vi "exp3p2.vi"() -> ()   [LabVIEW 2019]
uses:
  <vilib>/sound2/lvsound2.llb/Sound Data Format.ctl
  <vilib>/sound2/lvsound2.llb/Sampling Mode.ctl
  <vilib>/Analysis/2dsp.llb/Power Spectrum (DBL).vi
  <vilib>/sound2/lvsound2.llb/Sound Output Set Volume (Single).vi
  <vilib>/sound2/lvsound2.llb/Sound Output Write (DBL Single).vi
  <vilib>/Analysis/NI_AALPro.lvlib
panel:
  in  "sample mode":T1=1 items=["Finite Samples", "Continuous Samples"]
  in  "Volume":dbl(slide) scale=0.0..100.0
  in  "sound format":T2={"sample rate (S/s)"=22050.0, "number of channels"=2, "bits per sample"=16}
  in  "device ID":u32
  out "SNR (dB)":dbl
  out "Frequency Estimate (Hz)":dbl
  out "Frequency Domain Waveform":waveform(dbl)(graph)
  out "Time Domain Waveform":waveform(dbl)(graph)
  in  "Noise Std":dbl
  in  "Frequency Deviation (Hz)":dbl
  in  "stop":bool
  in  "Sampling Frequency":dbl
  in  "AWGN":bool
  in  "phase":dbl format="%0.2f"
  in  "frequency":dbl=1.0 format="%0.2f"
  in  "amplitude":dbl=1.0 format="%0.2f"
  in  "Frequency Hopping":bool
  in  "Number of Samples":i32
  in  "Square vs Sine":bool
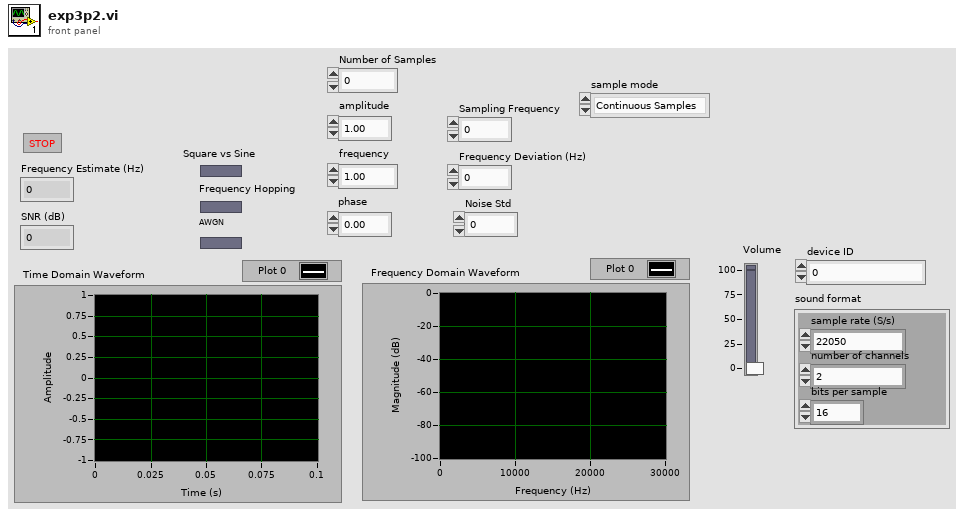
[diagram p1: front panel]
types:
  T1 = typedef "Sampling Mode.ctl" = i32
  T2 = typedef "Sound Data Format.ctl" = cluster{"sample rate (S/s)":dbl, "number of channels":i32, "bits per sample":i32}
  T3 = typedef "Sound Output Task ID.ctl" = u32
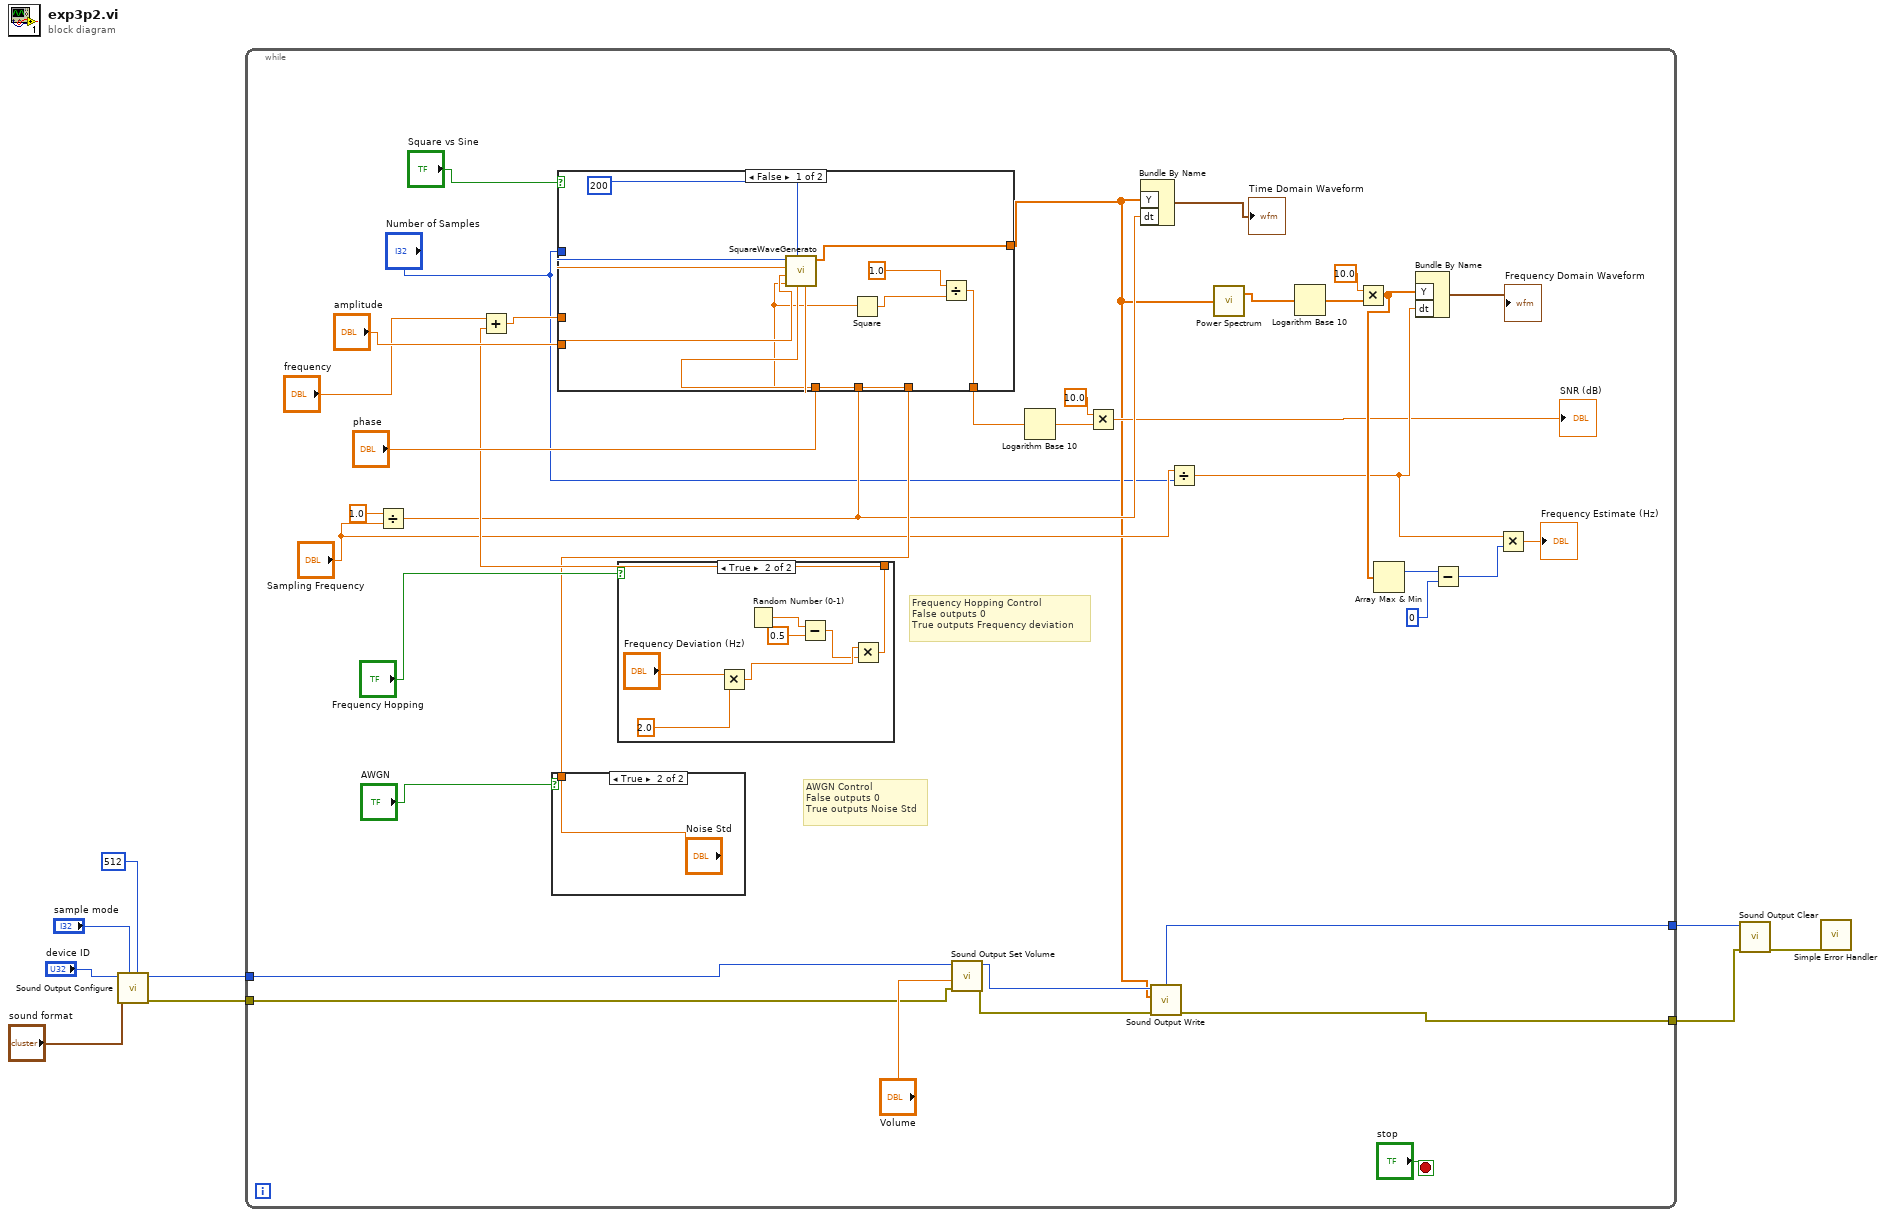
[diagram p0: block diagram]
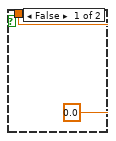
[diagram p2: hidden frame]
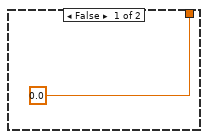
[diagram p3: hidden frame]
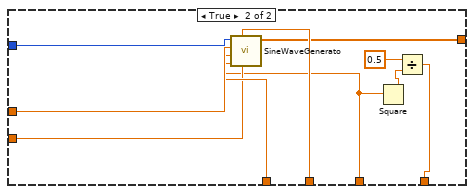
[diagram p4: hidden frame]
diagram:
  n1 = call <vilib>:"Sound Output Configure.vi"("number of samples/ch"=512, "sample mode"="sample mode", "sound format"="sound format", "device ID"="device ID") -> ("error out"=w2:errorcluster, "task ID"=w3:T3)  [unwired: 6 in]
  n2 = while {
    tunnel: [w15] -> w9
    tunnel: [w14] -> w8
    tunnel: w3 -> [w11]
    tunnel: w2 -> [w10]
    stop <- "stop" stop-if-true
    # "AWGN Control\nFalse outputs 0\nTrue outputs Noise Std"
    # "Frequency Hopping Control\nFalse outputs 0\nTrue outputs Frequency deviation"
    n3 = Divide(x=1.0, y="Sampling Frequency") -> (x/y=w35:dbl)
    n4 = case shown="True" "AWGN" {
      tunnel: [0.0 "Noise Std"] -> w36
      frame False {
      }
      frame True {
      }
    }
    n5 = case shown="True" "Frequency Hopping" {
      tunnel: [0.0 w50] -> w39
      frame False {
      }
      frame True {
        n6 = Multiply(x="Frequency Deviation (Hz)", y=2.0) -> (x*y=w52:dbl)
        n7 = Random Number (0-1)() -> (number: 0 to 1=w54:dbl)
        n8 = Subtract(x=w54, y=0.5) -> (x-y=w51:dbl)
        n9 = Multiply(x=w52, y=w51) -> (x*y=w50:dbl)
      }
    }
    n10 = Add(x="frequency", y=w39) -> (x+y=w37:dbl)
    n11 = case shown="False" "Square vs Sine" {
      tunnel: w35 -> [w66 w76]
      tunnel: w37 -> [w65 w75]
      tunnel: "Number of Samples" -> [w64 w77]
      tunnel: "phase" -> [w63 w74]
      tunnel: "amplitude" -> [w62 w73]
      tunnel: w36 -> [w60 w71]
      tunnel: [w61 w72] -> w16
      tunnel: [w57 w68] -> w20
      frame False {
        n12 = call "SquareWaveGenerato.vi"("Sampling Period"=w66, "phase"=w63, "Iteration Count"=200, "Noise Std"=w60, "amplitude"=w62, "frequency"=w65, "Number of Samples"=w64) -> ("Array"=w61:dbl[])  [unwired: 4 in]
        n13 = Square(x=w60) -> (x^2=w58:dbl)
        n14 = Divide(x=1.0, y=w58) -> (x/y=w57:dbl)
      }
      frame True {
        n15 = call "SineWaveGenerato.vi"("amplitude"=w73, "Sampling Period"=w76, "Noise Std"=w71, "phase"=w74, "frequency"=w75, "Number of Samples"=w77) -> ("Array"=w72:dbl[])  [unwired: 5 in]
        n16 = Square(x=w71) -> (x^2=w70:dbl)
        n17 = Divide(x=0.5, y=w70) -> (x/y=w68:dbl)
      }
    }
    n18 = call-poly <vilib>:"Sound Output Set Volume.vi"("error in (no error)"=w10, "volume"="Volume", "task ID"=w11) -> ("error out"=w17:errorcluster, "task ID out"=w18:T3)  [unwired: 7 in]
    n19 = Logarithm Base 10(1:w20) -> (0:w22:dbl)
    n20 = Multiply(x=10.0, y=w22) -> (x*y=→"SNR (dB)":dbl)
    n21 = Bundle By Name("Y"=w16, "dt"=w35) -> (→"Time Domain Waveform":waveform(dbl))  [unwired: 1 in]
    n22 = call-poly <vilib>:"Sound Output Write.vi"("error in (no error)"=w17, "data"=w16, "task ID"=w18) -> ("error out"=w14:errorcluster, "task ID out"=w15:T3)  [unwired: 7 in]
    n23 = Divide(x="Sampling Frequency", y="Number of Samples") -> (x/y=w24:dbl)
    n24 = call-poly <vilib>:"Power Spectrum.vi"("X"=w16) -> ("Power Spectrum"=w33:dbl[])  [unwired: 1 out]
    n25 = Logarithm Base 10(1:w33) -> (0:w32:dbl[])
    n26 = Multiply(x=10.0, y=w32) -> (x*y=w28:dbl[])
    n27 = Array Max & Min(array=w28) -> (max index (indices)=w27:i32)  [unwired: 3 out]
    n28 = Bundle By Name("Y"=w28, "dt"=w24) -> (→"Frequency Domain Waveform":waveform(dbl))  [unwired: 1 in]
    n29 = Subtract(x=w27, y=0) -> (x-y=w25:i32)
    n30 = Multiply(x=w24, y=w25) -> (x*y=→"Frequency Estimate (Hz)":dbl)
  }
  n31 = call <vilib>:"Sound Output Clear.vi"("error in (no error)"=w8, "task ID"=w9) -> ("error out"=w7:errorcluster)  [unwired: 9 in]
  n32 = call <vilib>:"Simple Error Handler.vi"("error in (no error)"=w7) -> ()  [unwired: 4 in, 5 out]
